vi "2_04.vi"() -> ()   [LabVIEW 2013]
panel:
  out "Salida":waveform(dbl)
  in  "Indice de bloques":dbl
  in  "Agudos":dbl
  in  "Medios":dbl
  in  "Bajos":dbl
  in  "Entrada":waveform(dbl)
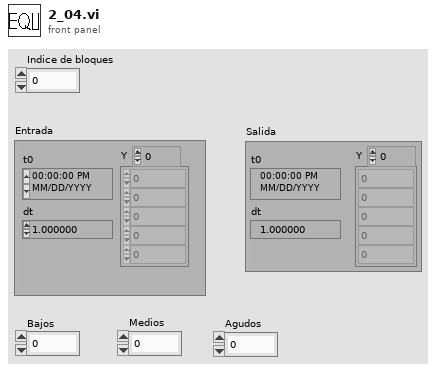
[diagram p1: front panel]
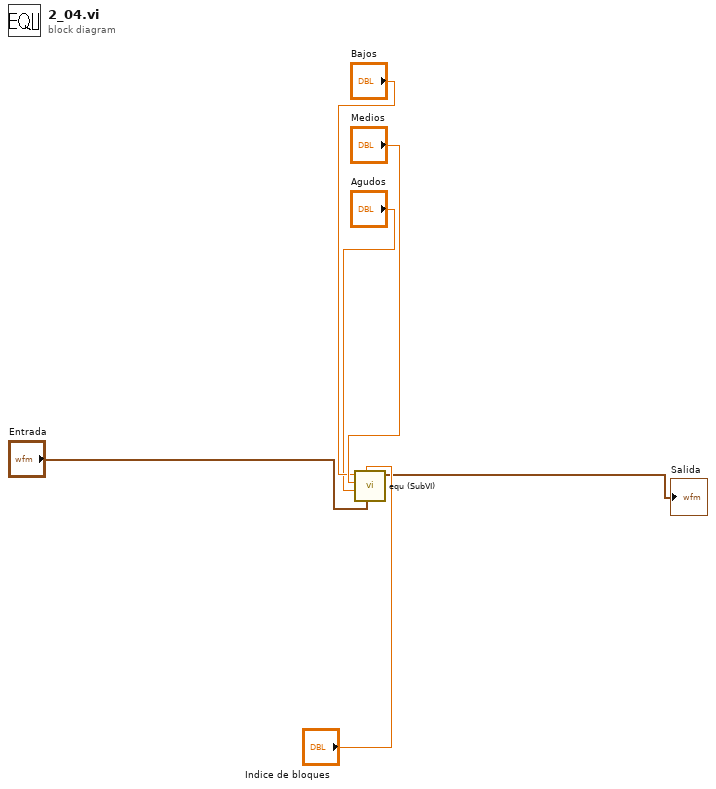
[diagram p0: block diagram]
diagram:
  n1 = call "equ (SubVI).vi"("Entrada"="Entrada", "Indice de bloques"="Indice de bloques", "Agudos"="Agudos", "Medios"="Medios", "Bajos"="Bajos") -> ("Salida"=→"Salida":waveform(dbl))  [unwired: 6 in]
